vi "Vision Processing.vi"(4 "error in (no error)":errorcluster) -> ()   [LabVIEW 2011]
doc: "This VI runs in parallel to other tasks. It gets images from the camera, processes them for color or shape and use that information to affect robot behavior."
uses:
  Robot Global Data.vi
  <vilib>/vision/NI_Vision_Development_Module.lvlib
panel:
  in  "Camera Name":string="Camera"
  in  "View 2":bool
  in  "Processing":enum32{"Color", "Intensity", "Intensity Open"}(tab)
  in  "Luminance":i32=255
  in  "Saturation":i32=255
  in  "Hue":i32(knob)=65 scale=0.0..255.0
  in  "Margins":cluster{"Hue":i32, "Sat":i32, "Lum":i32}={"Hue"=20, "Sat"=27, "Lum"=30} {"Sat" scale=0.0..40.0; "Lum" scale=0.0..40.0; "Hue" scale=0.0..40.0}
  in  "Range":cluster{"Lower value":sgl, "Upper value":sgl}={"Lower value"=150.0, "Upper value"=255.0} {"Lower value" scale=0.0..255.0; "Upper value" scale=0.0..255.0}
  in  "Range 2":cluster{"Lower value":sgl, "Upper value":sgl}={"Lower value"=150.0, "Upper value"=255.0} {"Lower value" scale=0.0..255.0; "Upper value" scale=0.0..255.0}
  in  "Particle Count Limit":i32=8
  in  "Area Size Limit":i32=444
  in  "Score Limits":T1={"Rect Coverage"=76.0, "Aspect Ratio"=70.0, "X Edge Strength"=40.0, "Y Edge Strength"=60.0}
  in  "Camera Type":enum16{"206", "1011"}(ring)
  out "Target Info":T2(array[cluster])
  in  "View":bool
  out "Original Image":T3(plugin-control)
  out "Processed Image":T3(plugin-control)
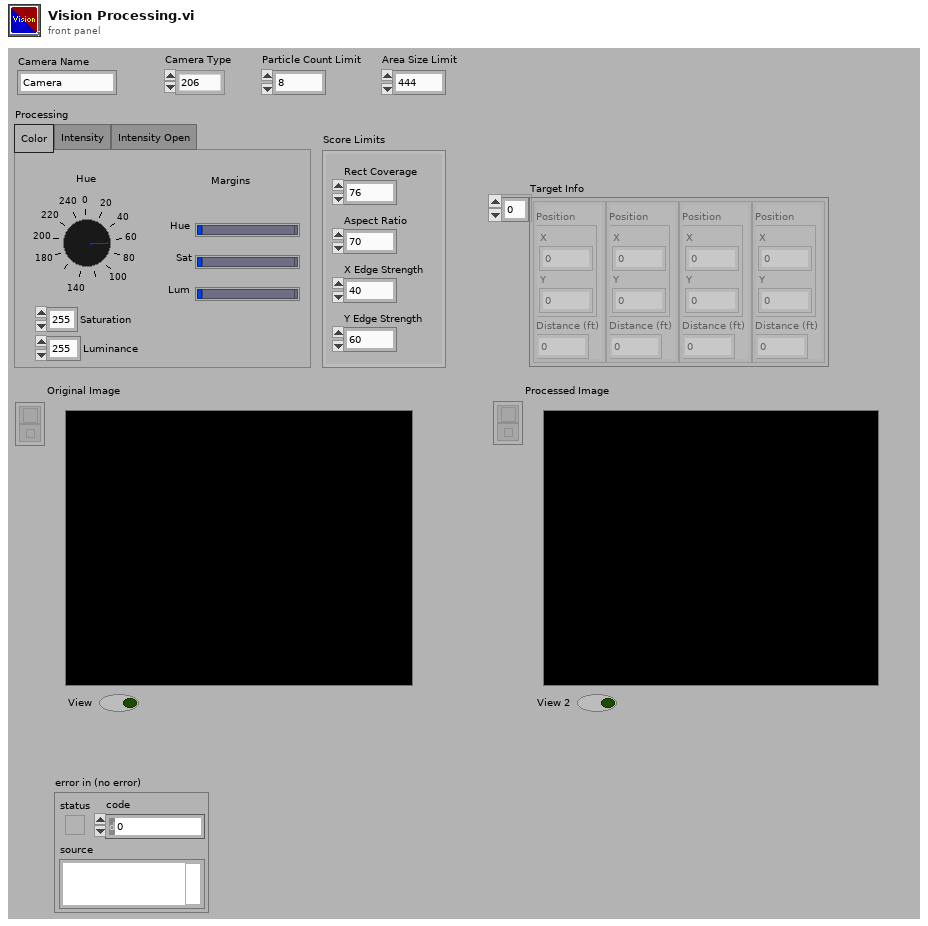
[diagram p1: front panel]
types:
  T1 = cluster{"Rect Coverage":dbl, "Aspect Ratio":dbl, "X Edge Strength":dbl, "Y Edge Strength":dbl}
  T2 = cluster{"Position":cluster{"X":dbl, "Y":dbl}, "Distance (ft)":dbl}[]
  T3 = typedef "IMAQ Image.ctl" = refnum<image>
  T4 = typedef "Image Type" = u32
  T5 = typedef "WPI_CameraDevRef.ctl" = cluster{"Camera Address":string, "CameraStatus":errorcluster, "Acquire Image Notifier":refnum<notifier>}
  T6 = enum32{"AutoM", "Close", "Dilate", "Erode", "Gradient", "Gradient out", "Gradient in", "Hit miss", "Open", "PClose", "POpen", "Thick", "Thin"}
  T7 = typedef "WPI_CameraImageSize.ctl" = enum16{"640x480", "320x240", "160x120"}
  T8 = cluster{cluster{"Left":dbl, "Top":dbl, "Right":dbl, "Bottom":dbl}, dbl[]}[]
  T9 = cluster{"Left":dbl, "Top":dbl, "Right":dbl, "Bottom":dbl}
  T10 = cluster{"Target Center (-1 to 1)":cluster{"X":dbl, "Y":dbl}, "Distance (ft)":dbl}
  T11 = cluster{"Target Center (-1 to 1)":cluster{"X":dbl, "Y":dbl}, "Distance (ft)":dbl}[]
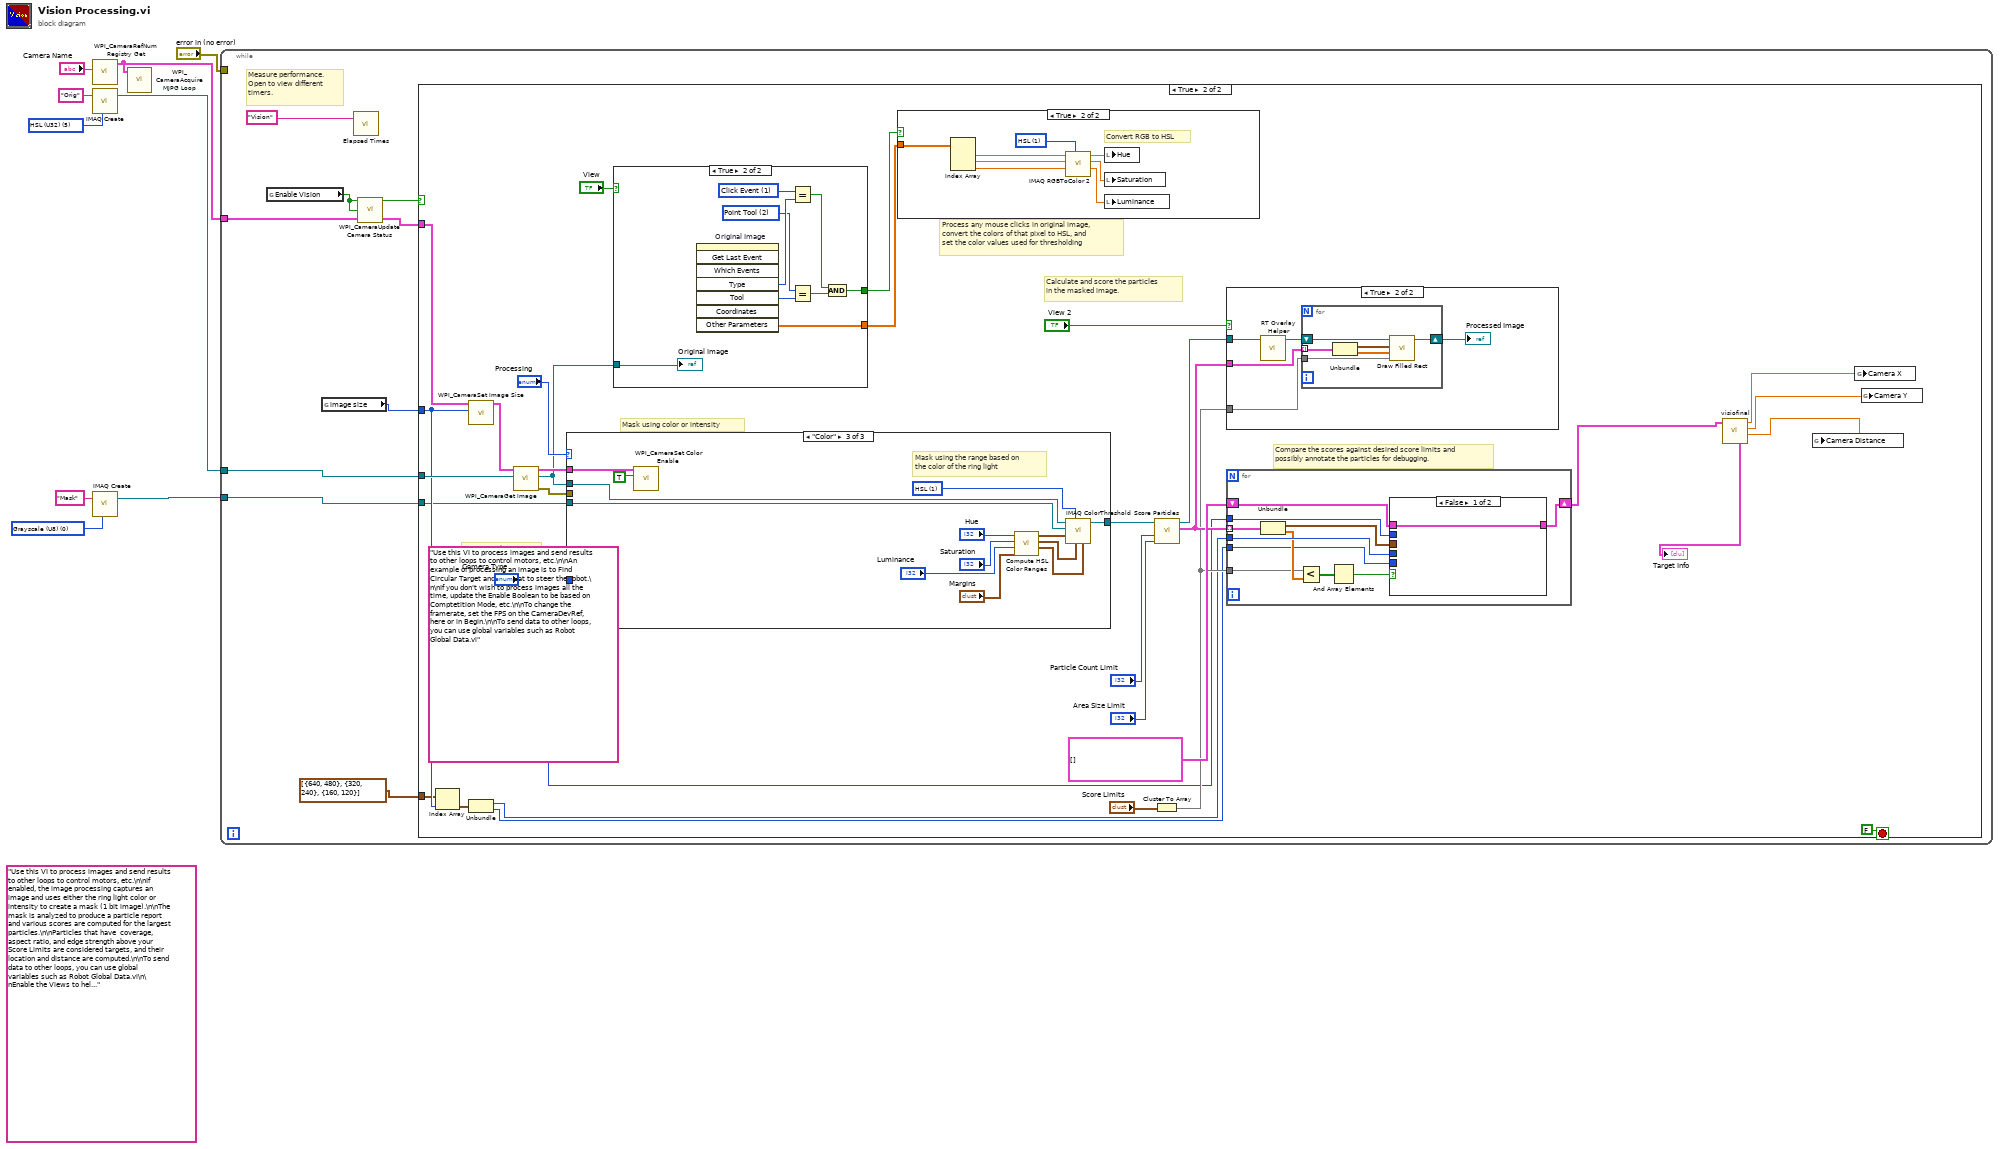
[diagram p0: block diagram]
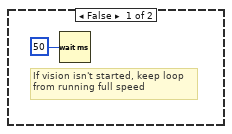
[diagram p2: hidden frame]
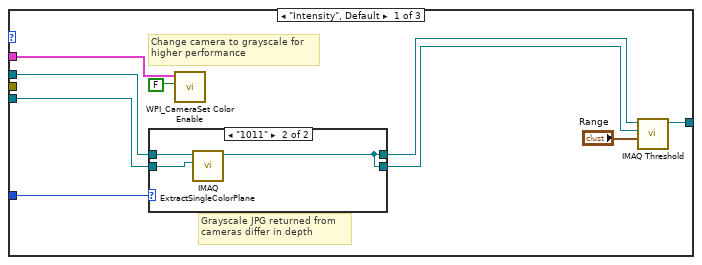
[diagram p4: hidden frame]
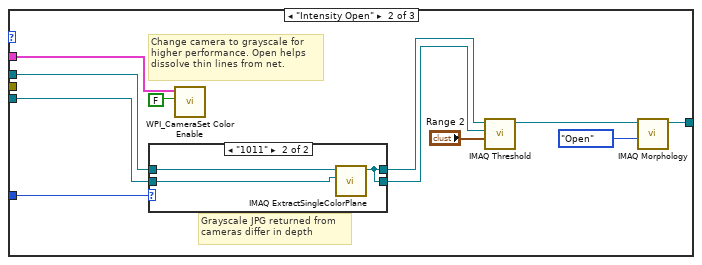
[diagram p6: hidden frame]
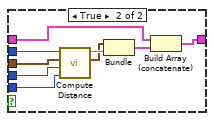
[diagram p10: hidden frame]
diagram:
  w3 = T4 0 items=["Grayscale (U8)", "Grayscale (I16)", "Grayscale (SGL)", "Complex (CSG)", "RGB (U32)", "HSL (U32)", "RGB (U64)", "Grayscale (U16)"] ("Image Type")
  (unwired) "Use this VI to process images and send results to other loops to control motors, etc.\n\nIf enabled, the image processing captures an image and uses either the ring light color or intensity to create a mask (1 bit image).\n\nThe mask is analyzed to produce a particle report and various scores are computed for the largest particles.\n\nParticles that have  coverage, aspect ratio, and edge strength above your Score Limits are considered targets, and their location and distance are computed.\n\nTo send data to other loops, you can use global variables such as Robot Global Data.vi\n\nEnable the Views to help debug color settings. Disable the View to speed up processing."
  w8 = T4 5 items=["Grayscale (U8)", "Grayscale (I16)", "Grayscale (SGL)", "Complex (CSG)", "RGB (U32)", "HSL (U32)", "RGB (U64)", "Grayscale (U16)"] ("Image Type")
  (unwired) "Use this VI to process images and send results to other loops to control motors, etc.\n\nAn example of processing an image is to Find Circular Target and use that to steer the robot.\n\nIf you don't wish to process images all the time, update the Enable Boolean to be based on Comptetition Mode, etc.\n\nTo change the framerate, set the FPS on the CameraDevRef, here or in Begin.\n\nTo send data to other loops, you can use global variables such as Robot Global Data.vi"
  n1 = call <vilib>:"WPI_CameraRefNum Registry Get.vi"("refnum name"="Camera Name") -> ("CameraDevRef"=w5:T5)  [unwired: 9 in, 1 out]
  n2 = call "IMAQ Create"("Image Name"="Orig", "Image Type"=w8) -> ("New Image"=w7:T3)  [unwired: 2 in, 2 out]
  n3 = call "IMAQ Create"("Image Name"="Mask", "Image Type"=w3) -> ("New Image"=w1:T3)  [unwired: 2 in, 2 out]
  n4 = call <vilib>:"WPI_CameraAcquire MJPG Loop.vi"("CameraDevRef"=w5) -> ()  [unwired: 11 in]
  n5 = while {
    tunnel: w7 -> [w17]
    tunnel: w5 -> [w16]
    tunnel: "error in (no error)" -> [_]
    tunnel: w1 -> [w11]
    stop <- FALSE stop-if-true
    # "Measure performance.\nOpen to view different\ntimers."
    n6 = global read "Robot Global Data.vi" "Enable Vision"() -> (w14:bool)
    n7 = global read "Robot Global Data.vi" "image size"() -> (w12:T7)
    n8 = call "Elapsed Times.vi"("Call Name"="Vision") -> ()  [unwired: 2 in, 1 out]
    n9 = call <vilib>:"WPI_CameraUpdate Camera Status.vi"("CameraDevRef In"=w16, "Enable Vision"=w14) -> ("CameraDevRef Out"=w15:T5)  [unwired: 3 in]
    n10 = case shown="True" w14 {
      tunnel: w17 -> [_ w41]
      tunnel: w15 -> [_ w37]
      tunnel: w12 -> [_ w32]
      tunnel: w11 -> [_ w27]
      tunnel: cluster{i32, i32}[] [{640, 480}, {320, 240}, {160, 120}] -> [_ w31]
      frame False {
        # "If vision isn't started, keep loop\nfrom running full speed"
        n11 = Wait (ms)(milliseconds to wait=u32 50) -> ()  [unwired: 1 out]
      }
      frame True {
        # "Compare the scores against desired score limits and\npossibly annotate the particles for debugging."
        # "Process any mouse clicks in original image,\nconvert the colors of that pixel to HSL, and\nset the color values used for thresholding"
        # "Calculate and score the particles\nin the masked image."
        # "Mask using color or intensity"
        # "Get original image"
        n12 = Index Array(array=w31, index=w32) -> (element=w28:cluster{i32, i32})
        n13 = call <vilib>:"WPI_CameraSet Image Size.vi"("Image Size"=w32, "CameraDevRef"=w37) -> ("CameraDevRef Out"=w38:T5)  [unwired: 8 in, 1 out]
        n14 = Unbundle(w28) -> (w30:i32, w29:i32)
        n15 = call <vilib>:"WPI_CameraGet Image.vi"("Image"=w41, "CameraDevRef"=w38) -> ("error out"=w39:errorcluster, "Image Out"=w26:T3, "CameraDevRef Out"=w40:T5)  [unwired: 7 in]
        n16 = case shown="\"Color\"" "Processing" {
          tunnel: w26 -> [w63 w75 w101]
          tunnel: [w66 w80 w100] -> w35
          tunnel: w40 -> [w64 w78 w91]
          tunnel: w39 -> [_ _ _]
          tunnel: w27 -> [w62 w76 w89]
          tunnel: "Camera Type" -> [w61 w77 _]
          frame "Intensity", Default {
            # "Grayscale JPG returned from\ncameras differ in depth"
            # "Change camera to grayscale for\nhigher performance"
            n17 = case shown="\"1011\"" w61 {
              tunnel: w63 -> [w69 w72]
              tunnel: w62 -> [w68 w71]
              tunnel: [w69 w70] -> w60
              tunnel: [w68 w70] -> w59
              frame "206", Default {
              }
              frame "1011" {
                n18 = call "IMAQ ExtractSingleColorPlane"("Image Dst"=w71, "Image Src"=w72) -> ("Image Dst Out"=w70:T3)  [unwired: 8 in, 1 out]
              }
            }
            n19 = call <vilib>:"WPI_CameraSet Color Enable.vi"("Color Enabled"=FALSE, "CameraDevRef"=w64) -> ()  [unwired: 8 in, 2 out]
            n20 = call "IMAQ Threshold"("Range"="Range", "Image Dst"=w59, "Image Src"=w60) -> ("Image Dst Out"=w66:T3)  [unwired: 3 in, 5 out]
          }
          frame "Intensity Open" {
            # "Grayscale JPG returned from\ncameras differ in depth"
            # "Change camera to grayscale for\nhigher performance. Open helps\ndissolve thin lines from net."
            n21 = case shown="\"1011\"" w77 {
              tunnel: w75 -> [w85 w88]
              tunnel: w76 -> [w84 w87]
              tunnel: [w85 w86] -> w74
              tunnel: [w84 w86] -> w73
              frame "206", Default {
              }
              frame "1011" {
                n22 = call "IMAQ ExtractSingleColorPlane"("Image Dst"=w87, "Image Src"=w88) -> ("Image Dst Out"=w86:T3)  [unwired: 8 in, 1 out]
              }
            }
            n23 = call <vilib>:"WPI_CameraSet Color Enable.vi"("Color Enabled"=FALSE, "CameraDevRef"=w78) -> ()  [unwired: 8 in, 2 out]
            n24 = call "IMAQ Threshold"("Range"="Range 2", "Image Dst"=w73, "Image Src"=w74) -> ("Image Dst Out"=w81:T3)  [unwired: 3 in, 5 out]
            n25 = call "IMAQ Morphology"("Operation"=T6."Open", "Image Src"=w81) -> ("Image Dst Out"=w80:T3)  [unwired: 8 in, 1 out]
          }
          frame "Color" {
            w99 = u16 1 items=["RGB", "HSL", "HSV", "HSI"] ("Color Mode")
            # "Mask using the range based on\nthe color of the ring light"
            n26 = call <vilib>:"WPI_CameraSet Color Enable.vi"("Color Enabled"=TRUE, "CameraDevRef"=w91) -> ()  [unwired: 8 in, 2 out]
            n27 = call "Compute HSL Color Ranges.vi"("Margins"="Margins", "Luminance"="Luminance", "Saturation"="Saturation", "Hue"="Hue") -> ("Lum Range"=w96:cluster{i32, i32}, "Sat Range"=w97:cluster{i32, i32}, "Hue Range"=w98:cluster{i32, i32})  [unwired: 5 in]
            n28 = call "IMAQ ColorThreshold"("Blue or Luma or Val or Inten Range"=w96, "Green or Sat Range"=w97, "Color Mode"=w99, "Red or Hue Range"=w98, "Image Dst"=w89, "Image Src"=w101) -> ("Image Dst Out"=w100:T3)  [unwired: 4 in, 1 out]
          }
        }
        n29 = case shown="True" "View" {
          tunnel: w26 -> [_ w121]
          tunnel: [_ w116] -> w34
          tunnel: [_ w113] -> w33
          frame False {
          }
          frame True {
            w114 = 2 items=["None", "Selection Tool", "Point Tool", "Line Tool", "Rectangle Tool", "Oval Tool", "Polygon Tool", "ClosedFreehandTool", "Annulus Tool", "Rotated Rectangle Tool", "Zoom Tool", "Pan Tool", "Polyline Tool", "Freehand Tool"] ("Tool")
            w115 = 1 items=["No Event"=0, "Click Event"=1, "Draw Event"=2, "Size Event"=4, "Scroll Event"=5, "Double Click Event"=8] ("Type")
            n30 = invoke on="Original Image" class="ImageControl" method="Get Last Event"() -> ("Type"=w117:i32, "Tool"=w120:i32, "Other Parameters"=w113:sgl[])  [unwired: 8 in, 5 out]
            n31 = Equal?(x=w115, y=w117) -> (x = y?=w118:bool)
            n32 = Equal?(x=w114, y=w120) -> (x = y?=w119:bool)
            n33 = And(x=w118, y=w119) -> (x .and. y?=w116:bool)
            "Original Image" <- w121
          }
        }
        n34 = case shown="True" w34 {
          tunnel: w33 -> [_ w58]
          frame False {
          }
          frame True {
            w57 = u16 1 items=["RGB", "HSL", "HSV", "HSI", "CIE L*a*b*", "CIE XYZ"] ("Color Mode")
            # "Convert RGB to HSL"
            n35 = Index Array(array=w58) -> (element #1=w56:sgl, element #2=w54:sgl, element #3=w52:sgl)  [unwired: 3 in]
            n36 = call "IMAQ RGBToColor 2"("Color Mode"=w57, "Blue value"=w52, "Green value"=w54, "Red value"=w56) -> ("Blue or Luma or Val or Inten or Z or b*value"=w51:dbl, "Green or Sat or Y or a* value"=w53:dbl, "Red or Hue or X or L* value"=w55:dbl)  [unwired: 4 in, 1 out]
            n37 = local write "Hue"(w55) -> ()
            n38 = local write "Saturation"(w53) -> ()
            n39 = local write "Luminance"(w51) -> ()
          }
        }
        n40 = Cluster To Array(cluster="Score Limits") -> (array=w44:dbl[])
        n41 = call "Score Particles.vi"("Area Size Limit"="Area Size Limit", "Particle Count Limit"="Particle Count Limit", "Image Refnum in"=w35) -> ("Scored Particle Info"=w46:T8, "Image Refnum out"=w49:T3)  [unwired: 7 in]
        n42 = case shown="True" "View 2" {
          tunnel: w49 -> [_ w103]
          tunnel: w46 -> [_ w105]
          tunnel: w44 -> [_ w104]
          frame False {
          }
          frame True {
            n43 = call "RT Overlay Helper.vi"("Refnum in"=w103) -> ("Refnum out"=w106:T3)  [unwired: 10 in]
            n44 = for {
              shift-right: [w111] -> w102
              shift-left: w106 -> [w112]
              tunnel: w105 -> [w108] mode=indexing
              tunnel: w104 -> [w107]
              n45 = Unbundle(w108) -> (w109:T9, w110:dbl[])
              n46 = call "Draw Filled Rect.vi"("Limits"=w107, "Scores"=w110, "Bounding Box"=w109, "image in"=w112) -> ("image out"=w111:T3)  [unwired: 7 in]
            }
            "Processed Image" <- w102
          }
        }
        n47 = for {
          shift-right: [w131] -> w24
          shift-left: T2 [] -> [w132]
          tunnel: w30 -> [w130]
          tunnel: w46 -> [w128] mode=indexing
          tunnel: w44 -> [w123]
          tunnel: "Camera Type" -> [w127]
          tunnel: w29 -> [w122]
          n48 = Unbundle(w128) -> (w129:T9, w124:dbl[])
          n49 = Less?(x=w123, y=w124) -> (x < y?=w126:bool[])
          n50 = And Array Elements(Boolean array=w126) -> (logical AND=w125:bool)
          n51 = case shown="False" w125 {
            tunnel: w132 -> [w133 w142]
            tunnel: [w133 w141] -> w131
            tunnel: w129 -> [_ w137]
            tunnel: w130 -> [_ w139]
            tunnel: w127 -> [_ w136]
            tunnel: w122 -> [_ w135]
            frame False {
            }
            frame True {
              n52 = call "Compute Distance.vi"("Y Image Resolution"=w135, "X Image Resolution"=w139, "Bounding Box"=w137, "Camera Type"=w136) -> ("Target Center (-1 to 1)"=w134:cluster{"X":dbl, "Y":dbl}, "Distance (ft)"=w138:dbl)  [unwired: 6 in]
              n53 = Bundle("Target Center (-1 to 1)"=w134, "Distance (ft)"=w138) -> (w140:T10)  [unwired: 1 in]
              n54 = Build Array (concatenate)(w142, w140) -> (w141:T11)
            }
          }
        }
        n55 = call "visiofinal.vi"("Array"=w24) -> ("Distance (ft)"=w20:dbl, "Y"=w22:dbl, "X"=w21:dbl, "Target Info"=→"Target Info":T2)  [unwired: 7 in]
        n56 = global write "Robot Global Data.vi" "Camera Distance"(w20) -> ()
        n57 = global write "Robot Global Data.vi" "Camera X"(w21) -> ()
        n58 = global write "Robot Global Data.vi" "Camera Y"(w22) -> ()
      }
    }
  }
